vi "Start Continuous Stream.vi"(8 "error in (no error)":errorcluster, 10 "stream index":i32, 11 "refnum in":refnum<k20>) -> (0 "error out":errorcluster, 3 "refnum out":refnum<k20>)   [LabVIEW 2015, in "niInstr Streaming v1 Host.lvlib"]
doc: "Activates the stream to operate indefinitely. The stream enters the Continuous state and will only autonomously leave the continuous state in response to an error state (such as a buffer underflow/overflow condition). A user should monitor the health of the transfer by either using Get Stream State.vi, or through the use of the Wait... functions available in the host API.\n\nWhen a user wishes to stop a continuous stream, they should use the appropriate API function to do so. This may be Clear Stream.vi or Stop Stream.vi. Consult the documentation of those VIs for more information.\n\n<B>Input Parameters</B>\n\n<B>error in (no error)</B> 'error in' can accept error information wired from VIs previously called. Use this information to decide if any functionality should be bypassed in the event of errors from other VIs.\n\nRight-click the 'error in' control on the front panel and select 'Explain Error' or 'Explain Warning' from the shortcut menu for more information about the error.\n\n<B>stream index</B> Selects which stream index this VI will interface to. This is the index number at the end of the host interface controls (0..7).\n\n<B>refnum in</B> Wire in the session obtained from Open FPGA Reference.\n\n<B>Output Parameters</B>\n\n<B>error out</B> contains error information. This output provides standard error out functionality.\n\n<B>refnum out</B> Copy of refnum in"
uses:
  <instrlib>/_niInstr/Streaming/v1/Host/niInstr Streaming v1 Host.lvlib
  <vilib>/Utility/error.llb/Error Cluster From Error Code.vi
  <vilib>/ErrorRing/Error Ring.xnode
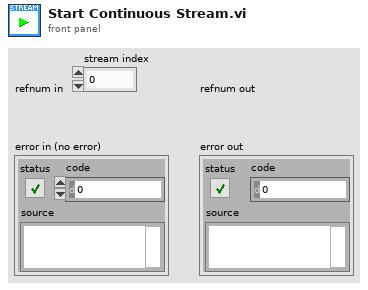
[diagram p1: front panel]
types:
  T1 = typedef "niInstr Streaming v1 Common.lvlib/Stream State.ctl" = enum8{"Idle", "Finite Transfer", "Continuous", "Done", "Error", "Not Ready", "Cancel"}
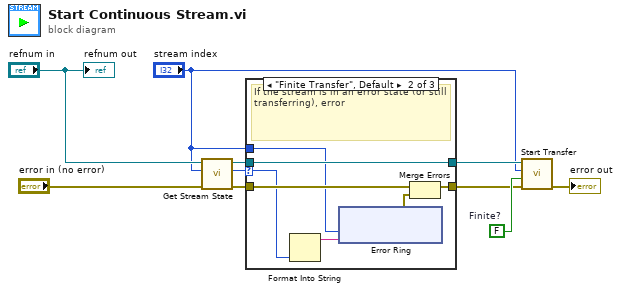
[diagram p0: block diagram]
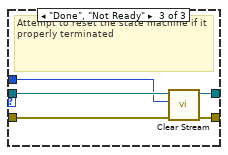
[diagram p3: hidden frame]
diagram:
  w8 = FALSE  # Finite?
  n1 = call <instrlib>:"Get Stream State.vi"("error in (no error)"="error in (no error)", "stream index"="stream index", "refnum in"="refnum in") -> ("error out"=w6:errorcluster, "stream state"=w2:T1, "refnum out"=w3:refnum<k20>)  [unwired: 6 in]
  n2 = case shown="\"Finite Transfer\", Default" w2 {
    selector: w2 -> [_ w15 _]
    tunnel: w3 -> [w12 w19 w31]
    tunnel: w6 -> [w11 w17 w32]
    tunnel: "stream index" -> [_ w13 w30]
    tunnel: [w12 w19 w29] -> w4
    tunnel: [w11 w16 w28] -> w5
    frame "Idle" {
      # "If the state machine is already idle, it then it is safe to resume"
    }
    frame "Finite Transfer", Default {
      # "If the stream is in an error state (or still transferring), error"
      n3 = Format Into String(w15) -> (resulting string=w14:string)  [unwired: 3 in, 1 out]
      n4 = xnode "Error Ring"("parameter 0"=w13, "parameter 1"=w14) -> ("error out"=w18:errorcluster)
      n5 = Merge Errors(w17, w18) -> (w16:errorcluster)
    }
    frame "Done", "Not Ready" {
      # "Attempt to reset the state machine if it properly terminated"
      n6 = call <instrlib>:"Clear Stream.vi"("error in (no error)"=w32, "stream index"=w30, "refnum in"=w31) -> ("error out"=w28:errorcluster, "refnum out"=w29:refnum<k20>)  [unwired: 7 in]
    }
  }
  n7 = call <instrlib>:"Start Transfer.vi"("error in (no error)"=w5, "finite?"=w8, "stream index"="stream index", "refnum in"=w4) -> ("error out"=→"error out":errorcluster)  [unwired: 6 in, 1 out]
  "refnum out" <- "refnum in"
